vi "Update_Data.vi"(8 "error in (no error)":errorcluster caption="entrée d'erreur (pas d'erreur)", 11 "Firebase AssembledProducts P1817 en entrée":refnum<class "Firebase AssembledProducts P1817.lvclass">) -> (0 "error out":errorcluster caption="sortie d'erreur", 3 "Firebase AssembledProducts P1817 en sortie":refnum<class "Firebase AssembledProducts P1817.lvclass">)   [LabVIEW 2020, in "Library Instrument & Equipement.lvlib" / "Library FireBase.lvlib" / "Firebase AssembledProducts P1817.lvclass"]
doc: "Create New document\nPlease initialise the following values\n - Name BDD\n - Document\n - API Key"
uses:
  Firebase AssembledProducts P1817.lvclass
  C:/Users/ngarcin/OneDrive - Altyor/Standard TB/Class/Firebase/Source/Firebase Driver/Firebase Driver.lvclass
  Firebase AssembledProducts P1817.lvclass/Firebase AssembledProducts P1817.ctl
  Firebase Altyor/Firebase Altyor.lvclass
  Firebase Driver/Firebase Driver.lvclass
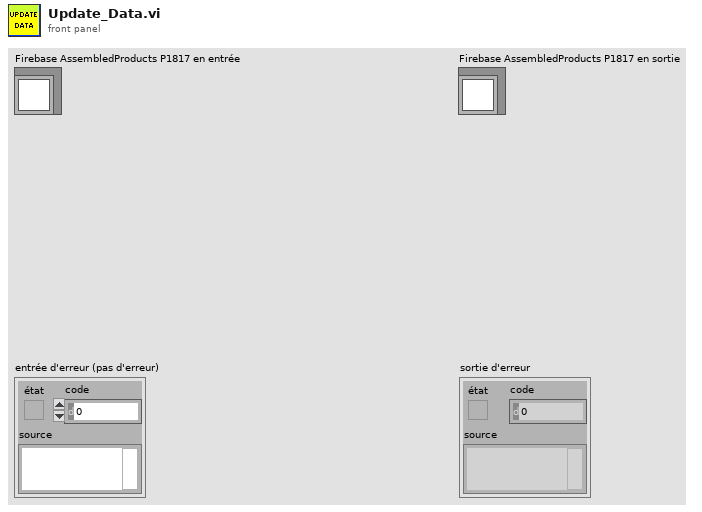
[diagram p1: front panel]
types:
  T1 = cluster{"fields":cluster{"Result":cluster{"booleanValue":bool}, "CreationDate":cluster{"timestampValue":string}, "Batch":cluster{"stringValue":string}, "SerialNumber":cluster{"stringValue":string}, "EndOfProduction":cluster{"timestampValue":string}, "FW_Version":cluster{"mapValue":cluster{"fields":cluster{"Bootloader":cluster{"mapValue":cluster{"fields":cluster{"File_Name":cluster{"stringValue":string}, "Version":cluster{"mapValue":cluster{"fields":cluster{"Major":cluster{"stringValue":string}, "Minor":cluster{"stringValue":string}}}}, "Checksum":cluster{"stringValue":string}}}}, "SoftDevice":cluster{"mapValue":cluster{"fields":cluster{"File_Name":cluster{"stringValue":string}, "Version":cluster{"mapValue":cluster{"fields":cluster{"Major":cluster{"stringValue":string}, "Minor":cluster{"stringValue":string}}}}, "Checksum":cluster{"stringValue":string}}}}, "DFU":cluster{"mapValue":cluster{"fields":cluster{"File_Name":cluster{"stringValue":string}, "Version":cluster{"mapValue":cluster{"fields":cluster{"Major":cluster{"stringValue":string}, "Minor":cluster{"stringValue":string}}}}, "Checksum":cluster{"stringValue":string}}}}}}}, "PartNumber":cluster{"stringValue":string}, "OrderNumber":cluster{"stringValue":string}, "Operator":cluster{"stringValue":string}, "AssembledProductName":cluster{"stringValue":string}, "Delivery":cluster{"booleanValue":bool}}}
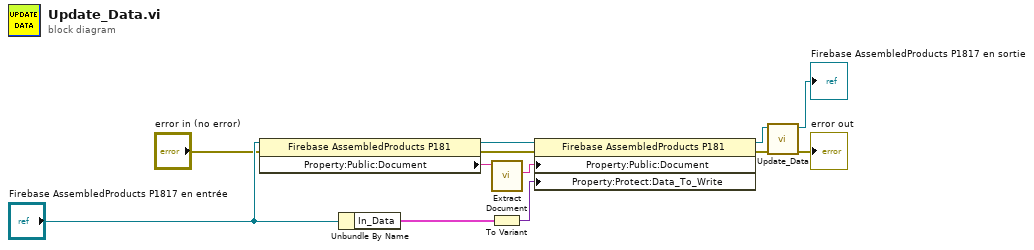
[diagram p0: block diagram]
diagram:
  n1 = property class="Firebase AssembledProducts P181"(reference="Firebase AssembledProducts P1817 en entrée", error in="error in (no error)") -> (reference out=w3:refnum<class "Firebase AssembledProducts P1817.lvclass">, error out=w1:errorcluster, "Property:Public:Document"=w6:string)
  n2 = Unbundle By Name("Firebase AssembledProducts P1817 en entrée") -> ("In_Data"=w8:T1)
  n3 = call "Extract Document.vi"("Name"=w6) -> ("Source"=w5:string)  [unwired: 9 in, 1 out]
  n4 = To Variant(anything=w8) -> (Variant=w7:variant)
  n5 = property class="Firebase AssembledProducts P181"(reference=w3, error in=w1, "Property:Public:Document"=w5, "Property:Protect:Data_To_Write"=w7) -> (reference out=w10:refnum<class "Firebase AssembledProducts P1817.lvclass">, error out=w9:errorcluster)
  n6 = call-parent "Update_Data.vi"("error in (no error)"=w9, "Firebase Altyor en entrée"=w10) -> ("error out"=→"error out":errorcluster, "Firebase Altyor en sortie"=→"Firebase AssembledProducts P1817 en sortie":refnum<class "Firebase AssembledProducts P1817.lvclass">)  [unwired: 8 in]
